vi "waitStatusSweepingStopped.vi"(8 "error in (no error)":errorcluster, 10 "time (s) [10 s]":dbl=10.0, 11 "Instrument.LockinAPI in":refnum<class "Instrument.LockinAPI.lvclass">) -> (0 "error out":errorcluster, 3 "Instrument.LockinAPI out":refnum<class "Instrument.LockinAPI.lvclass">)   [LabVIEW 2019, in "Instrument.LockinAPI.lvclass"]
uses:
  Instrument.LockinAPI.lvclass
  Typedefs/LockinAPI.getState.states--enum.ctl
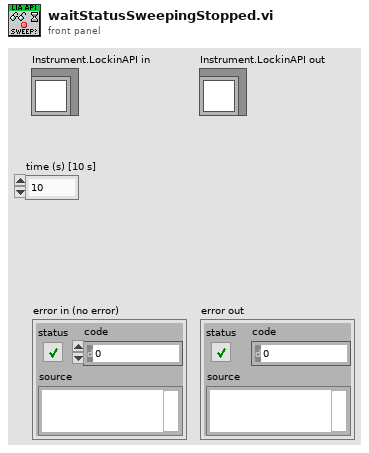
[diagram p1: front panel]
types:
  T1 = typedef "Instrument.LockinAPI.lvclass/LockinAPI.getState.states--enum.ctl" = enum16{"idle", "created", "started", "stopped", "sweeping"}
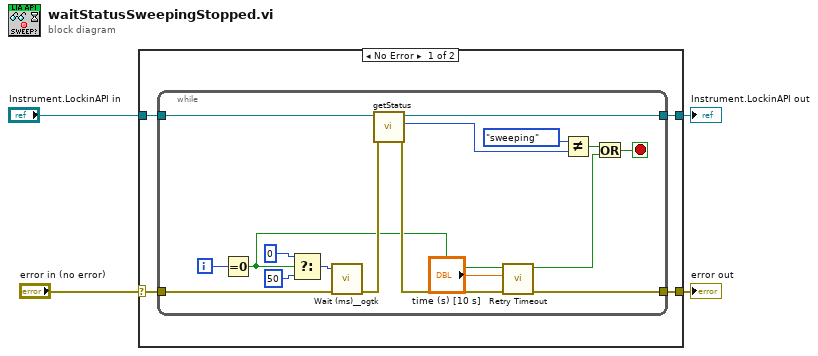
[diagram p0: block diagram]
diagram:
  n1 = case shown="No Error" "error in (no error)" {
    selector: "error in (no error)" -> [w5 w26]
    tunnel: [w8 w26] -> w4
    tunnel: [w7 w27] -> w3
    tunnel: "Instrument.LockinAPI in" -> [w6 w27]
    frame No Error {
      n2 = while {
        tunnel: w5 -> [w25]
        tunnel: [w15] -> w8
        tunnel: w6 -> [w20]
        tunnel: [w19] -> w7
        i -> [w13]
        stop <- w24 stop-if-true
        n3 = Equal To 0?(x=w13) -> (x = 0?=w12:bool)
        n4 = Select(t=u32 0, s=w12, f=u32 50 ("milliseconds to wait")) -> (s? t:f=w21:u32)
        n5 = call <userlib>:"Wait (ms)__ogtk.vi"("error in (no error)"=w25, "milliseconds to wait"=w21) -> ("error out"=w16:errorcluster)  [unwired: 8 in, 1 out]
        n6 = call-dynamic "getStatus.vi"("error in (no error)"=w16, "Instrument.LockinAPI in"=w20) -> ("error out"=w14:errorcluster, "state"=w18:T1, "Instrument.LockinAPI out"=w19:refnum<class "Instrument.LockinAPI.lvclass">)  [unwired: 7 in]
        n7 = call "Retry Timeout.vi"("error in (no error)"=w14, "time (s) [10 s]"="time (s) [10 s]", "reset"=w12) -> ("error out"=w15:errorcluster, "Timeout?"=w11:bool)  [unwired: 7 in]
        n8 = Not Equal?(x=LockinAPI.getState.states--enum."sweeping" ("state"), y=w18) -> (x != y?=w17:bool)
        n9 = Or(x=w17, y=w11) -> (x .or. y?=w24:bool)
      }
    }
    frame Error {
    }
  }
  "error out" <- w4
  "Instrument.LockinAPI out" <- w3
